vi "SubVIuPpercase2ndcharacter.vi"(1 "substring":string, 2 "string":string) -> (0 "result string":string)   [LabVIEW 2015]
doc: "Input\n1) string - the second character is going to replace with Uppercase of substring (2)\n2)substring - the second character is going to be Uppercased and replace the second character of string(1)\n\nOutput\n1)result string - result string that contains the edited string with the second Uppercase character"
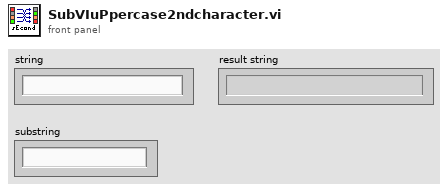
[diagram p1: front panel]
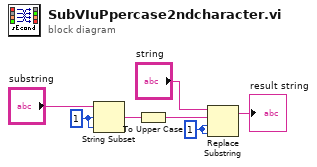
[diagram p0: block diagram]
diagram:
  w3 = 1 ("offset (0)")
  w4 = 1 ("offset (0)")
  n1 = String Subset(string="substring", offset (0)=w3, length (rest)=w3) -> (substring=w1:string)
  n2 = To Upper Case(1:w1) -> (0:w7:string)
  n3 = Replace Substring(2:w4, 3:w4, 4:w7, 5:"string") -> (1:→"result string":string)  [unwired: 1 out]
